vi "LabVIEW_Adq_Dades_v0.vi"() -> ()   [LabVIEW 2019]
uses:
  <vilib>/Analysis/NI_AALPro.lvlib
  <vilib>/Analysis/5stat.llb/RMS (DBL).vi
  <vilib>/Waveform/WDTOps.llb/WDT Index Channel DBL.vi
panel:
  in  "Botó d'abortar":bool
  in  "Botó de marxa":bool
  in  "Número de dades per fer mitjana":dbl
  in  "Interval entre dues adquisicions (ms)":dbl
  in  "Durada de l'adquisició (ms)":dbl
  in  "Número de canals a adquirir":dbl
  out "rms value":dbl format="%0.2f"
  out "t0":timestamp
  out "dt":dbl
  out "Waveform Graph 2":waveform(dbl)(graph)
  out "Valor actual":dynamicdata(graph)
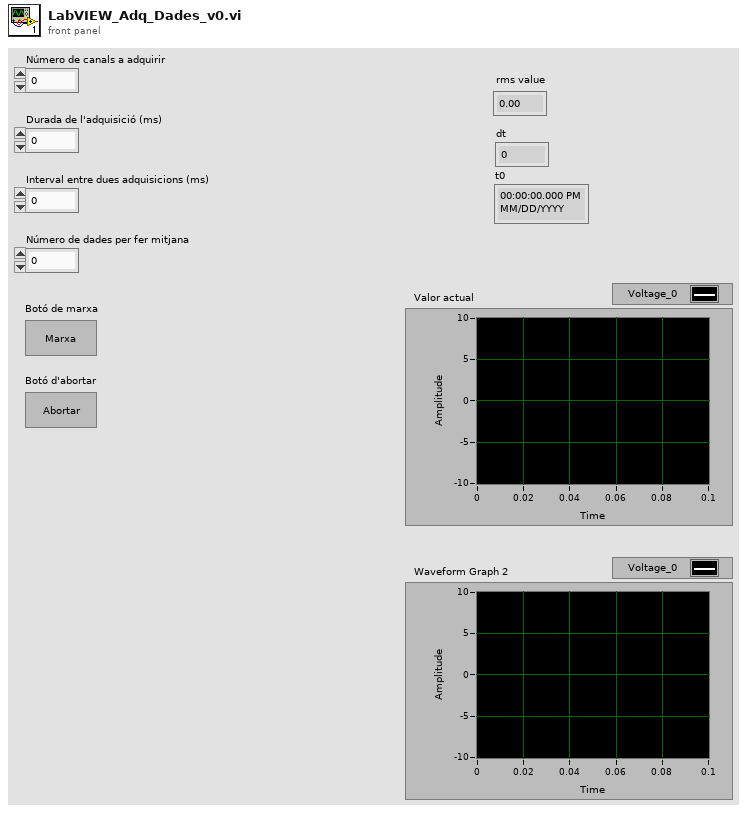
[diagram p1: front panel]
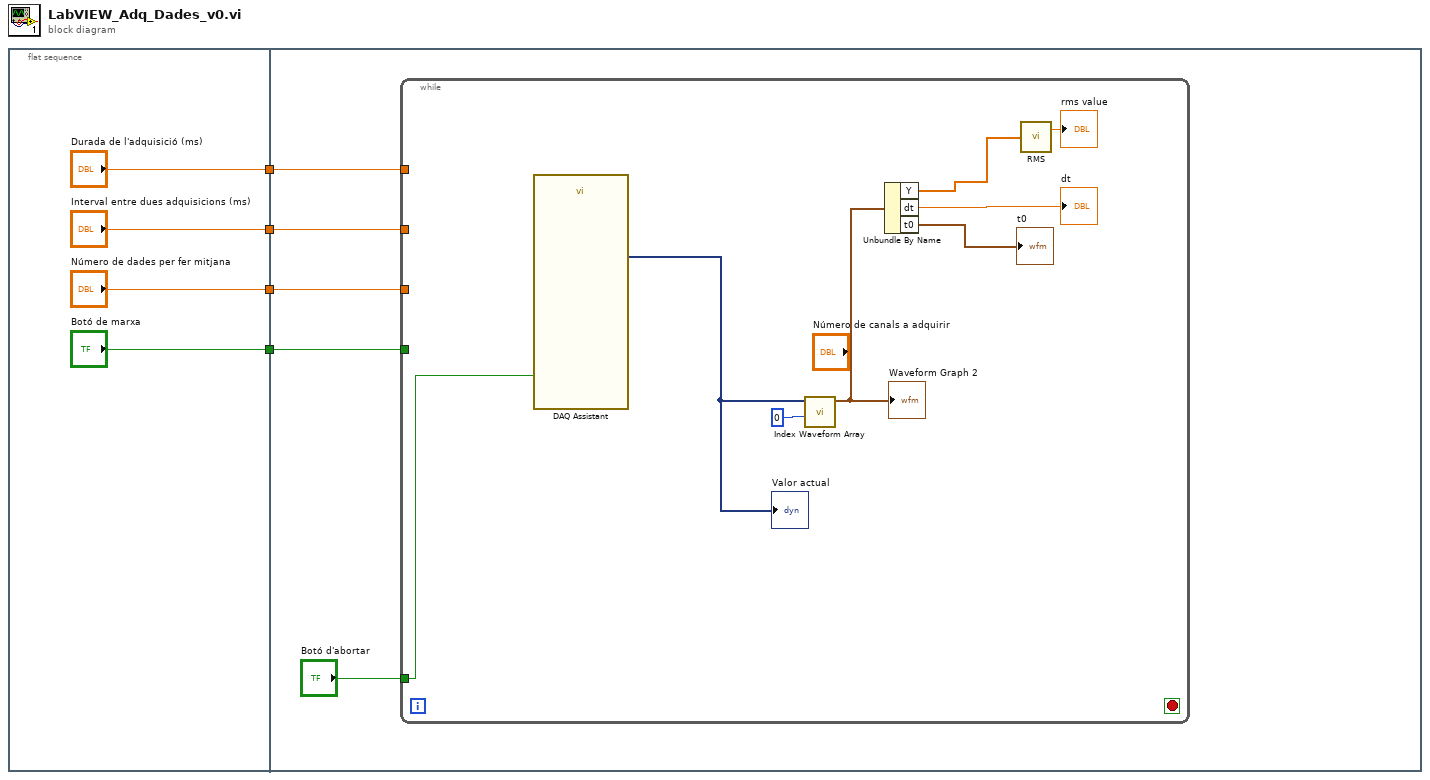
[diagram p0: block diagram]
diagram:
  n1 = flat-sequence {
    tunnel: ["Durada de l'adquisició (ms)"] -> w4
    tunnel: ["Interval entre dues adquisicions (ms)"] -> w3
    tunnel: ["Número de dades per fer mitjana"] -> w2
    tunnel: ["Botó de marxa"] -> w1
    tunnel: w4 -> [w13]
    tunnel: w3 -> [w12]
    tunnel: w2 -> [w11]
    tunnel: w1 -> [w10]
    frame #0 {
    }
    frame #1 {
      n2 = while {
        tunnel: w13 -> [_]
        tunnel: w12 -> [_]
        tunnel: w11 -> [_]
        tunnel: w10 -> [_]
        tunnel: "Botó d'abortar" -> [w14]
        stop <- _ stop-if-true
        n3 = call "DAQ Assistant"("stop (T)"=w14) -> ("data"=w16:dynamicdata)  [unwired: 16 in, 2 out]
        "Valor actual" <- w16
        n4 = call-poly <vilib>:"Index Waveform Array.vi"("index"=0, "waveform array"=w16) -> ("waveform"=w17:waveform(dbl))  [unwired: 8 in, 1 out]
        "Waveform Graph 2" <- w17
        n5 = Unbundle By Name(w17) -> ("Y"=w20:dbl[], "dt"=→"dt":dbl, "t0"=→"t0":timestamp)
        n6 = call-poly <vilib>:"RMS.vi"("X"=w20) -> ("rms value"=→"rms value":dbl)  [unwired: 1 out]
      }
    }
  }
